vi "FeedbackDecode_BuildStimCmd.vi"(2 "EncodeClustIn":T1={"ParamsTable"=[], "Sel"=[], "Stim"=FALSE, "StimMode"=enum."Off", "StimStep"=[enum."1uA", enum."1uA", enum."Off"], "Jitter"=FALSE, "Pulse"=FALSE, "BFreq"=0.0, "BAmp"=0.0, "UEAArray"=[], "AdjClust"={"Add"=FALSE, "Sub"=FALSE, "Val"=[1.0, 100.0, 0.2, 500.0, 0.0], "B"=[FALSE, FALSE, FALSE, FALSE, FALSE], "Inc+"=["x+1", "x+10", "x+0.1", "x+10", "x+10"], "Set"=FALSE, "LoadTable"=FALSE, "SaveTable"=FALSE, "ClearTable"=FALSE, "DeleteSel"=FALSE, "Inc-"=["x-1", "x-10", "x-0.1", "x-10", "x-10"]}, "PresetTable"=[], "SelPreset"=[], "SortClust"={"Region"=FALSE, "Receptor"=FALSE, "Electrode"=FALSE, "Min Amp"=FALSE, "Max Amp"=FALSE, "Min Freq"=FALSE, "Max Freq"=FALSE, "Duration"=FALSE}, "SelSort"={"Sel"=FALSE}, "PresetClust"={"Load"=FALSE, "Clear"=FALSE, "Save"=FALSE, "Del"=FALSE}, "RespClust"={"RespType"=enum."Sensor Map", "OpenResp"=FALSE}, "AmpLimit"=0.0, "FreqLimit"=0.0, "DurLimit"=0.0, "Wait Period"=0.0, "Train Period"=0.0} {"Train Period" min=0.0 max=100.0 step=0.1; "Wait Period" min=0.0 max=100.0 step=0.1; "DurLimit" min=0.0 max=1.0 step=0.01; "FreqLimit" min=0.0 max=500.0 step=1.0; "AmpLimit" min=0.0 max=100.0 step=1.0; "BAmp" min=0.0 max=100.0 step=1.0; "BFreq" min=0.0 max=100.0 step=1.0}) -> (0 "EncodeClustOut":T1={"ParamsTable"=[], "Sel"=[], "Stim"=FALSE, "StimMode"=enum."Off", "StimStep"=[enum."1uA", enum."1uA", enum."Off"], "Jitter"=FALSE, "Pulse"=FALSE, "BFreq"=0.0, "BAmp"=0.0, "UEAArray"=[], "AdjClust"={"Add"=FALSE, "Sub"=FALSE, "Val"=[1.0, 100.0, 0.2, 500.0, 0.0], "B"=[FALSE, FALSE, FALSE, FALSE, FALSE], "Inc+"=["x+1", "x+10", "x+0.1", "x+10", "x+10"], "Set"=FALSE, "LoadTable"=FALSE, "SaveTable"=FALSE, "ClearTable"=FALSE, "DeleteSel"=FALSE, "Inc-"=["x-1", "x-10", "x-0.1", "x-10", "x-10"]}, "PresetTable"=[], "SelPreset"=[], "SortClust"={"Region"=FALSE, "Receptor"=FALSE, "Electrode"=FALSE, "Min Amp"=FALSE, "Max Amp"=FALSE, "Min Freq"=FALSE, "Max Freq"=FALSE, "Duration"=FALSE}, "SelSort"={"Sel"=FALSE}, "PresetClust"={"Load"=FALSE, "Clear"=FALSE, "Save"=FALSE, "Del"=FALSE}, "RespClust"={"RespType"=enum."Sensor Map", "OpenResp"=FALSE}, "AmpLimit"=0.0, "FreqLimit"=0.0, "DurLimit"=0.0, "Wait Period"=0.0, "Train Period"=0.0} {"Train Period" min=0.0 max=100.0 step=0.1; "Wait Period" min=0.0 max=100.0 step=0.1; "DurLimit" min=0.0 max=1.0 step=0.01; "FreqLimit" min=0.0 max=500.0 step=1.0; "AmpLimit" min=0.0 max=100.0 step=1.0; "BAmp" min=0.0 max=100.0 step=1.0; "BFreq" min=0.0 max=100.0 step=1.0}, 1 "StimCmd":string)   [LabVIEW 2020]
uses:
  FeedbackDecode_EncodeClust.ctl
  FeedbackDecode_VariablesToString_Array.vi
  FeedbackDecode_VariablesToString_Scalar.vi
panel:
  in  "Receptor":string[](array[string])=["MS1", "MS2", "SA1", "RA1", "RA2", "aSA", "aRA", "scaled", "bio amp", "bio freq", "proprio"]
  in  "Region":string[](array[string])=["thumb_distal", "thumb_medial", "thumb_proximal", "index_distal", "index_medial", "index_proximal", "middle_distal", "middle_medial", "middle_proximal", "ring_distal", "ring_medial", "ring_proximal", "pinky_distal", "pinky_medial", "pinky_proximal", "palm_back", "palm_side", "palm_pinky", "palm_thumb", "thumb_MCP", "thumb_PIP", "thumb_DIP", "thumb_ABD", "index_MCP", "index_ABD", "middle_MCP", "ring_MCP", "pinky_MCP", "pinky_ABD", "wrist_FLEX", "wrist_UDEV", "wrist_PRO"]
  # "Value"
  # "Inc-"
  # "Inc+"
  # "Min Amp"
  # "Max Amp"
  # "Min Freq"
  # "Max Freq"
  # "Duration"
  # "Value"
  # "Inc-"
  # "Inc+"
  # "Min Amp"
  # "Max Amp"
  # "Min Freq"
  # "Max Freq"
  # "Duration"
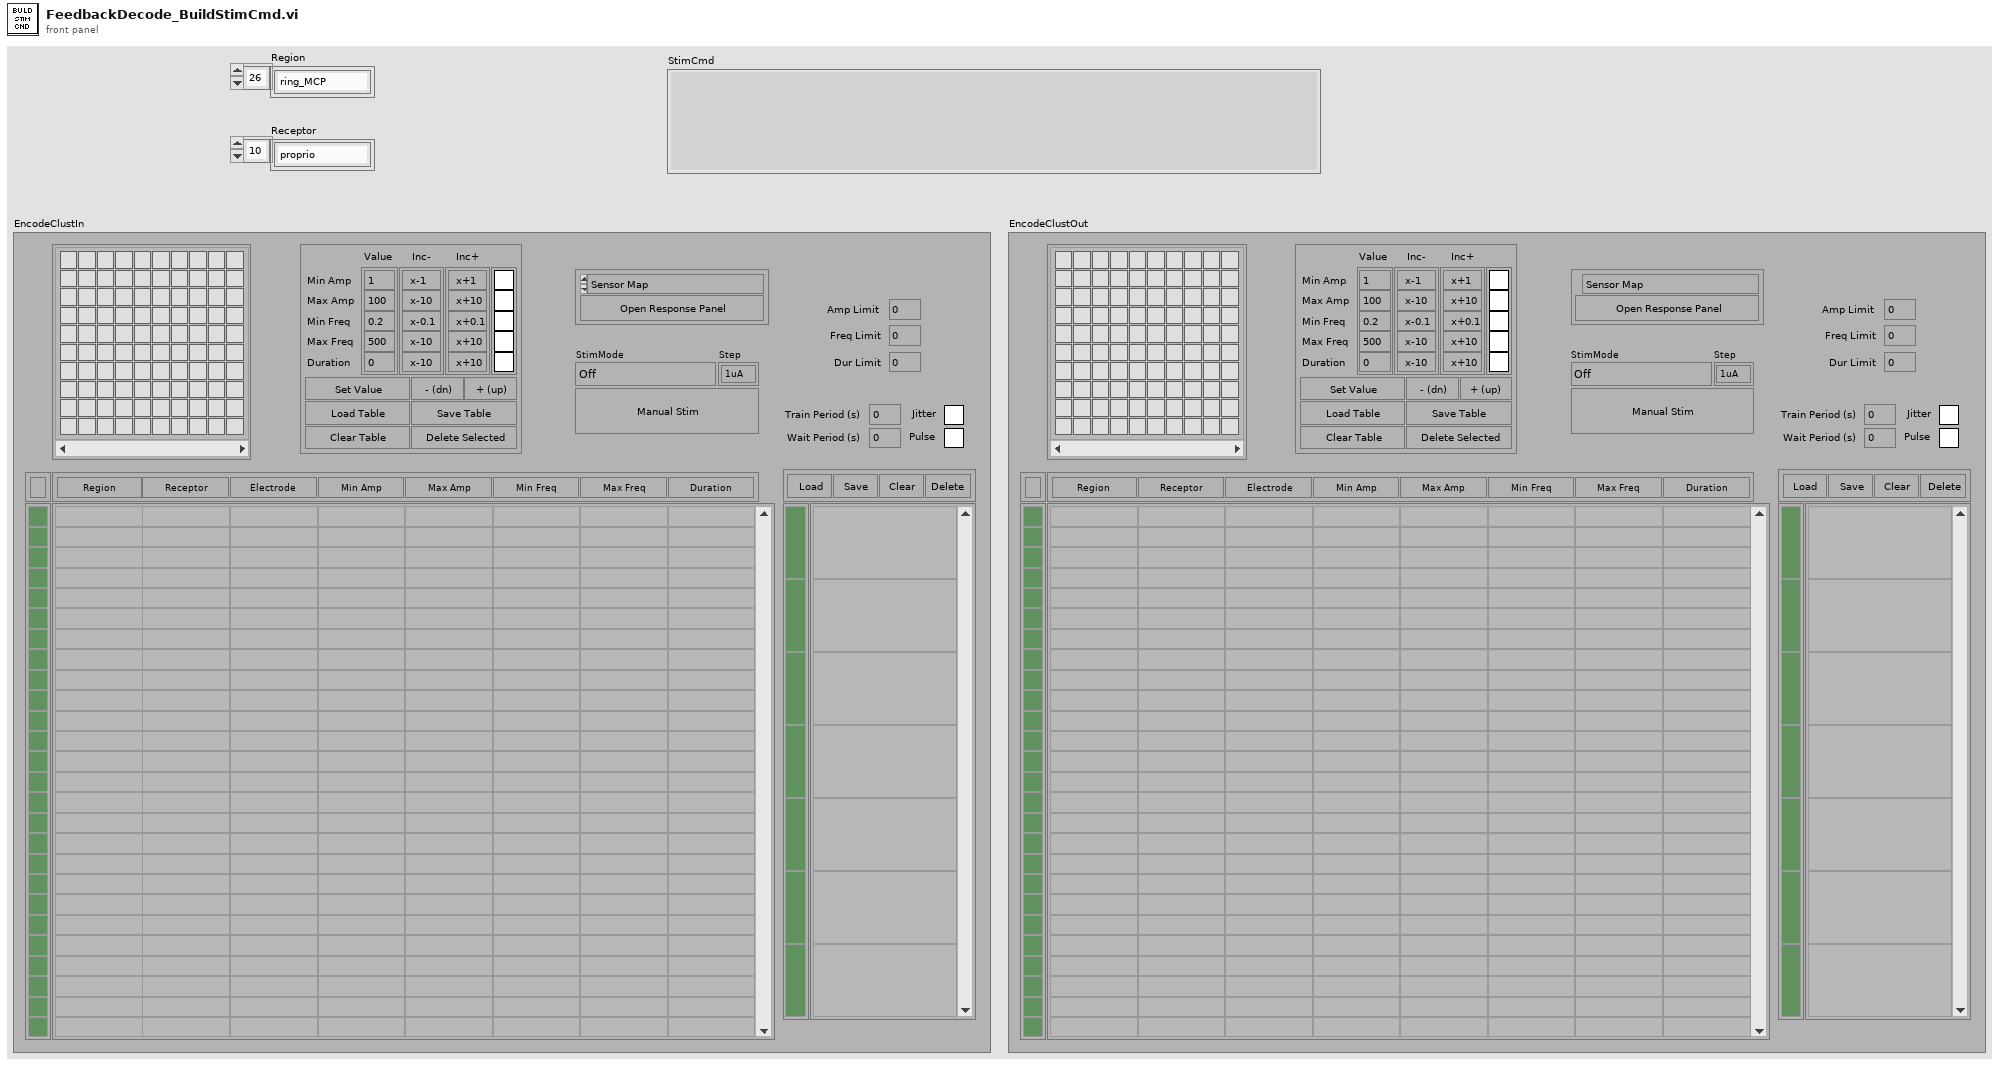
[diagram p1: front panel]
types:
  T1 = typedef "FeedbackDecode_EncodeClust.ctl" = cluster{"ParamsTable":string[][], "Sel":bool[], "Stim":bool, "StimMode":enum16{"Off", "Manual", "MSMS", "VRE", "3DHand", "DEKA", "Analog(DEKA)"}, "StimStep":enum16{"Off", "1uA", "2uA", "5uA", "10uA", "20uA", "30uA"}[], "Jitter":bool, "Pulse":bool, "BFreq":dbl, "BAmp":dbl, "UEAArray":cluster{"Boolean 1":bool, "Boolean 2":bool, "Boolean 3":bool, "Boolean 4":bool, "Boolean 5":bool, "Boolean 6":bool, "Boolean 7":bool, "Boolean 8":bool, "Boolean 9":bool, "Boolean 10":bool, "Boolean 11":bool, "Boolean 12":bool, "Boolean 13":bool, "Boolean 14":bool, "Boolean 15":bool, "Boolean 16":bool, "Boolean 17":bool, "Boolean 18":bool, "Boolean 19":bool, "Boolean 20":bool, "Boolean 21":bool, "Boolean 22":bool, "Boolean 23":bool, "Boolean 24":bool, "Boolean 25":bool, "Boolean 26":bool, "Boolean 27":bool, "Boolean 28":bool, "Boolean 29":bool, "Boolean 30":bool, "Boolean 31":bool, "Boolean 32":bool, "Boolean 33":bool, "Boolean 34":bool, "Boolean 35":bool, "Boolean 36":bool, "Boolean 37":bool, "Boolean 38":bool, "Boolean 39":bool, "Boolean 40":bool, "Boolean 41":bool, "Boolean 42":bool, "Boolean 43":bool, "Boolean 44":bool, "Boolean 45":bool, "Boolean 46":bool, "Boolean 47":bool, "Boolean 48":bool, "Boolean 49":bool, "Boolean 50":bool, "Boolean 51":bool, "Boolean 52":bool, "Boolean 53":bool, "Boolean 54":bool, "Boolean 55":bool, "Boolean 56":bool, "Boolean 57":bool, "Boolean 58":bool, "Boolean 59":bool, "Boolean 60":bool, "Boolean 61":bool, "Boolean 62":bool, "Boolean 63":bool, "Boolean 64":bool, "Boolean 65":bool, "Boolean 66":bool, "Boolean 67":bool, "Boolean 68":bool, "Boolean 69":bool, "Boolean 70":bool, "Boolean 71":bool, "Boolean 72":bool, "Boolean 73":bool, "Boolean 74":bool, "Boolean 75":bool, "Boolean 76":bool, "Boolean 77":bool, "Boolean 78":bool, "Boolean 79":bool, "Boolean 80":bool, "Boolean 81":bool, "Boolean 82":bool, "Boolean 83":bool, "Boolean 84":bool, "Boolean 85":bool, "Boolean 86":bool, "Boolean 87":bool, "Boolean 88":bool, "Boolean 89":bool, "Boolean 90":bool, "Boolean 91":bool, "Boolean 92":bool, "Boolean 93":bool, "Boolean 94":bool, "Boolean 95":bool, "Boolean 96":bool, "Boolean 97":bool, "Boolean 98":bool, "Boolean 99":bool, "Boolean 100":bool}[], "AdjClust":cluster{"Add":bool, "Sub":bool, "Val":dbl[], "B":bool[], "Inc+":string[], "Set":bool, "LoadTable":bool, "SaveTable":bool, "ClearTable":bool, "DeleteSel":bool, "Inc-":string[]}, "PresetTable":string[][], "SelPreset":bool[], "SortClust":cluster{"Region":bool, "Receptor":bool, "Electrode":bool, "Min Amp":bool, "Max Amp":bool, "Min Freq":bool, "Max Freq":bool, "Duration":bool}, "SelSort":cluster{"Sel":bool}, "PresetClust":cluster{"Load":bool, "Clear":bool, "Save":bool, "Del":bool}, "RespClust":cluster{"RespType":enum16{"Sensor Map", "Full Map"}, "OpenResp":bool}, "AmpLimit":dbl, "FreqLimit":dbl, "DurLimit":dbl, "Wait Period":dbl, "Train Period":dbl}
  T2 = enum16{"Off", "Manual", "MSMS", "VRE", "3DHand", "DEKA", "Analog(DEKA)"}
  T3 = enum16{"Off", "1uA", "2uA", "5uA", "10uA", "20uA", "30uA"}[]
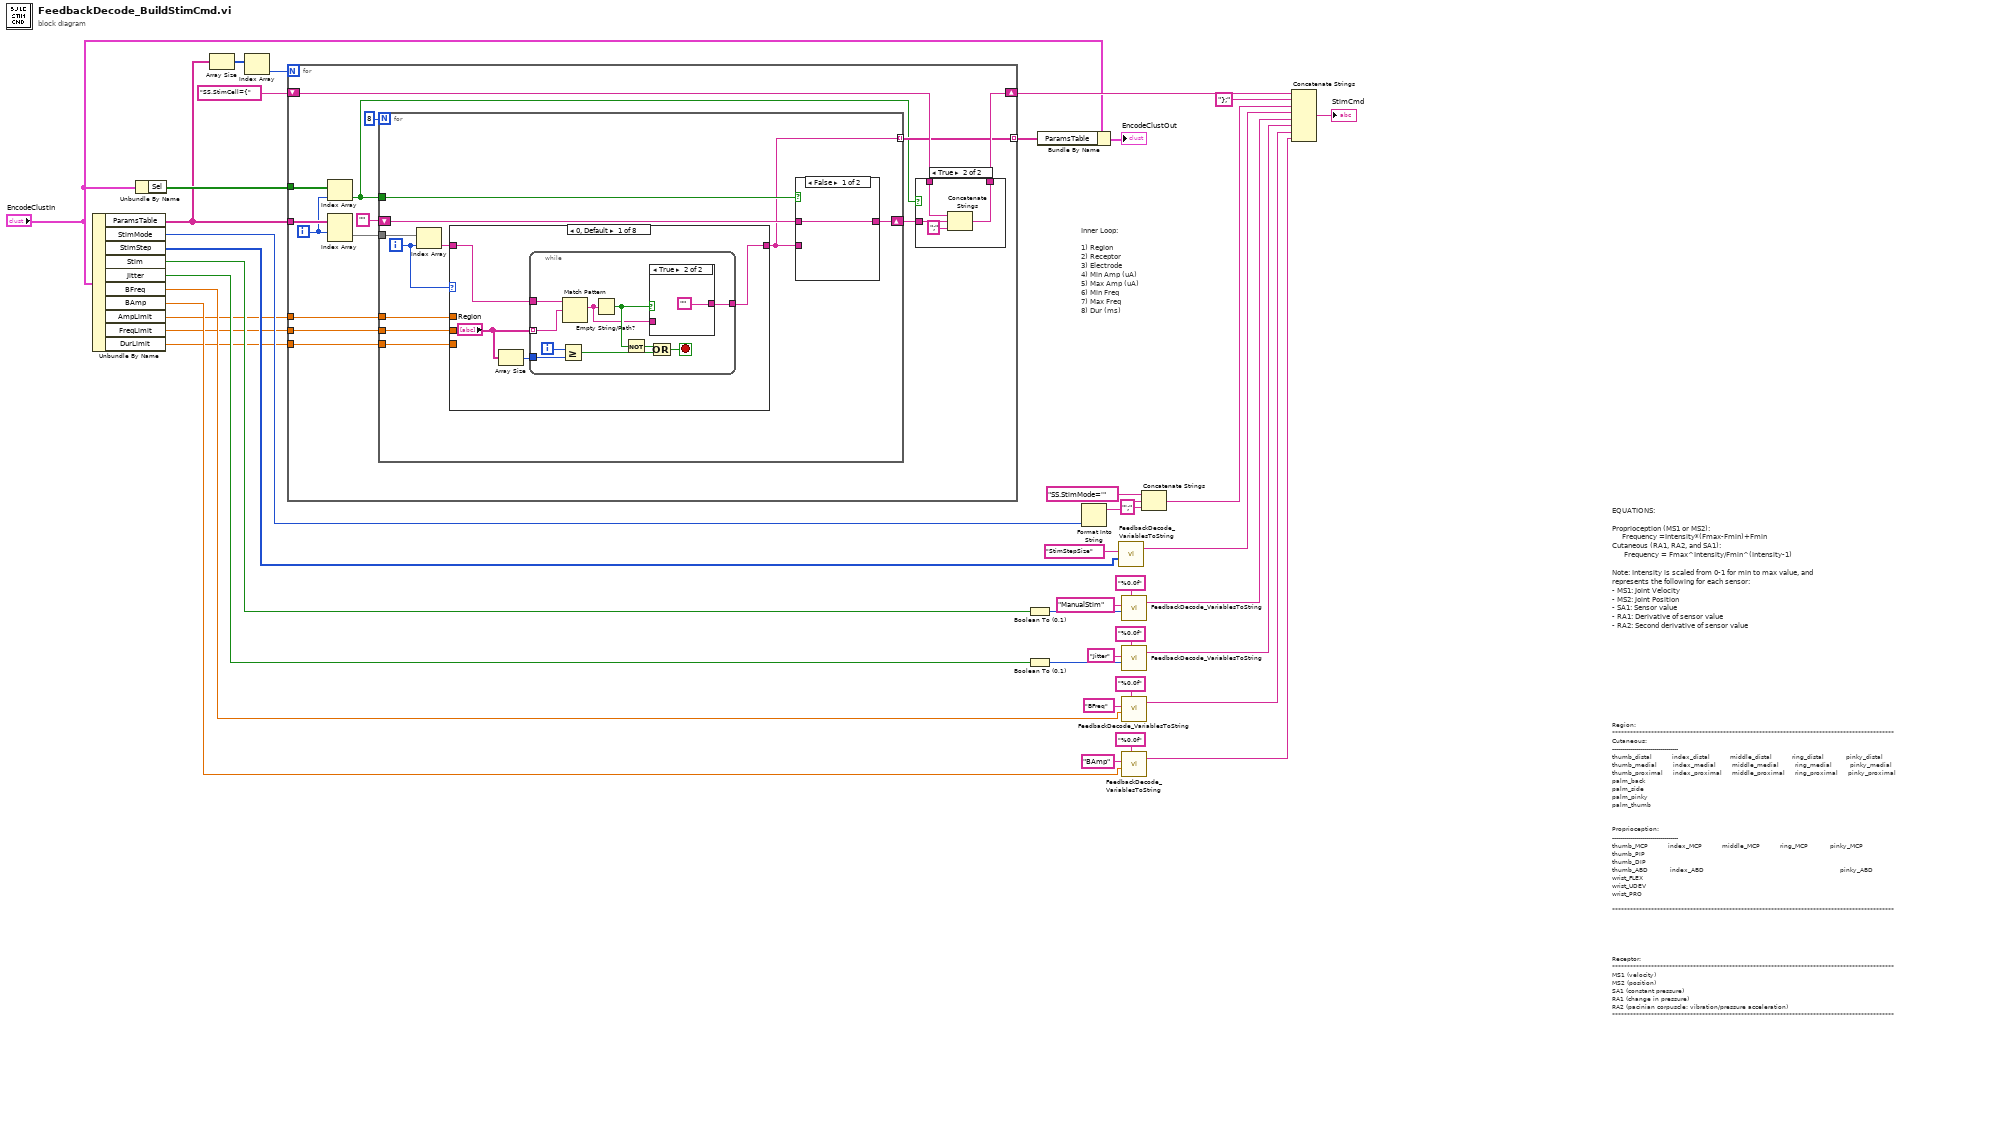
[diagram p0: block diagram]
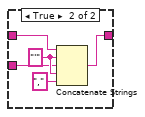
[diagram p3: hidden frame]
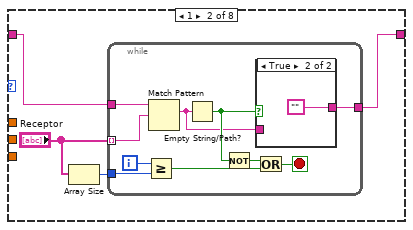
[diagram p5: hidden frame]
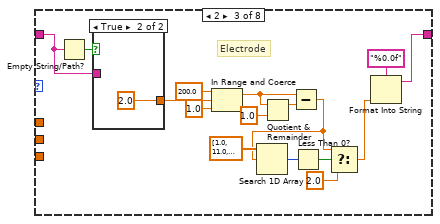
[diagram p7: hidden frame]
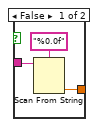
[diagram p8: hidden frame]
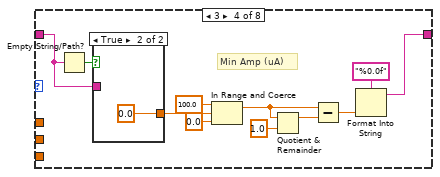
[diagram p9: hidden frame]
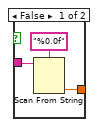
[diagram p10: hidden frame]
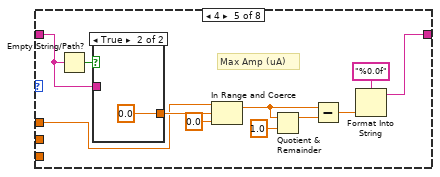
[diagram p11: hidden frame]
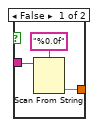
[diagram p12: hidden frame]
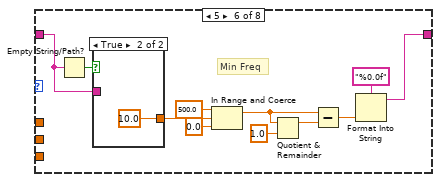
[diagram p13: hidden frame]
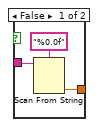
[diagram p14: hidden frame]
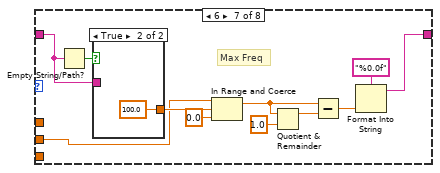
[diagram p15: hidden frame]
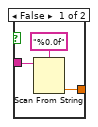
[diagram p16: hidden frame]
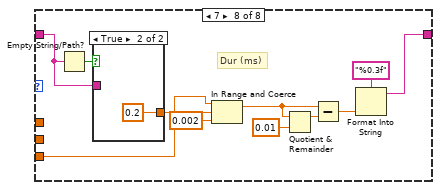
[diagram p17: hidden frame]
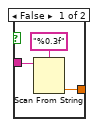
[diagram p18: hidden frame]
diagram:
  # "Inner Loop:\n\n1) Region\n2) Receptor\n3) Electrode\n4) Min Amp (uA)\n5) Max Amp (uA)\n6) Min Freq\n7) Max Freq\n8) Dur (ms)"
  # "EQUATIONS:\n\nProprioception (MS1 or MS2):\n     Frequency =Intensity*(Fmax-Fmin)+Fmin\nCutaneous (RA1, RA2, and SA1):     \n      Frequency = Fmax^Intensity/Fmin^(Intensity-1)\n\nNote: Intensity is scaled from 0-1 for min to max value, and represents the following for each sensor:\n- MS1: Joint Velocity\n- MS2: Joint Position\n- SA1: Sensor value\n- RA1: Derivative of sensor value\n- RA2: Second derivative of sensor value"
  # "Region:\n**********************************************************************************************\nCutaneous:\n---------------------------------\nthumb_distal          index_distal          middle_distal          ring_distal           pinky_distal\nthumb_medial        index_medial        middle_medial        ring_medial         pinky_medial\nthumb_proximal     index_proximal     middle_proximal     ring_proximal     pinky_proximal\npalm_back\npalm_side\npalm_pinky\npalm_thumb\n\n\nProprioception:\n---------------------------------\nthumb_MCP          index_MCP          middle_MCP          ring_MCP           pinky_MCP\nthumb_PIP                          \nthumb_DIP                                   \nthumb_ABD           index_ABD                                                                    pinky_ABD\nwrist_FLEX\nwrist_UDEV\nwrist_PRO\n\n**********************************************************************************************\n\n\n\n\n\nReceptor:\n**********************************************************************************************\nMS1 (velocity)\nMS2 (position)\nSA1 (constant pressure)\nRA1 (change in pressure)\nRA2 (pacinian corpuscle: vibration/pressure acceleration)\n**********************************************************************************************"
  n1 = Unbundle By Name("EncodeClustIn") -> ("ParamsTable"=w34:string[][], "StimMode"=w27:T2, "StimStep"=w26:T3, "Stim"=w18:bool, "Jitter"=w13:bool, "BFreq"=w9:dbl, "BAmp"=w5:dbl, "AmpLimit"=w3:dbl, "FreqLimit"=w2:dbl, "DurLimit"=w1:dbl)
  n2 = Unbundle By Name("EncodeClustIn") -> ("Sel"=w40:bool[])
  n3 = Array Size(array=w34) -> (size(s)=w33:i32[])
  n4 = Index Array(array=w33) -> (element=w32:i32)  [unwired: 1 in]
  n5 = for {
    N: w32 -> [_]
    tunnel: w40 -> [w46]
    tunnel: w34 -> [w48]
    shift-right: [w53] -> w39
    shift-left: "SS.StimCell={" -> [w54]
    tunnel: [w47] -> w36 mode=indexing
    tunnel: w3 -> [w43]
    tunnel: w2 -> [w42]
    tunnel: w1 -> [w41]
    i -> [w45]
    n6 = Index Array(array=w46, index=w45) -> (element=w44:bool)
    n7 = Index Array(array=w48, index (row)=w45) -> (element=w51:string[])  [unwired: 1 in]
    n8 = for {
      N: 8 -> [_]
      tunnel: w51 -> [w69]
      shift-right: [w67] -> w49
      shift-left: "" -> [w68]
      tunnel: w44 -> [w65]
      tunnel: [w63] -> w47 mode=indexing
      tunnel: w43 -> [w62]
      tunnel: w42 -> [w61]
      tunnel: w41 -> [w60]
      i -> [w64]
      n9 = Index Array(array=w69, index=w64) -> (element=w66:string)
      n10 = case shown="0, Default" w64 {
        tunnel: w66 -> [w79 w94 w114 w129 w145 w159 w175 w189]
        tunnel: [w78 w93 w116 w128 w144 w158 w174 w190] -> w63
        tunnel: w62 -> [_ _ _ _ w143 _ _ _]
        tunnel: w61 -> [_ _ _ _ _ _ w173 _]
        tunnel: w60 -> [_ _ _ _ _ _ _ w188]
        frame 0, Default {
          n11 = Array Size(array="Region") -> (size(s)=w77:i32)
          n12 = while {
            tunnel: "Region" -> [w88] mode=indexing
            tunnel: w79 -> [w89]
            tunnel: [w80] -> w78
            tunnel: w77 -> [w87]
            i -> [w86]
            stop <- w83 stop-if-true
            n13 = Greater Or Equal?(x=w86, y=w87) -> (x >= y?=w84:bool)
            n14 = Match Pattern(string=w89, regular expression=w88) -> (match substring=w81:string)  [unwired: 1 in, 3 out]
            n15 = Empty String/Path?(string/path=w81) -> (empty?=w82:bool)
            n16 = Not(x=w82) -> (.not. x?=w85:bool)
            n17 = case shown="True" w82 {
              tunnel: w81 -> [w90 _]
              tunnel: [w90 ""] -> w80
              frame False {
              }
              frame True {
              }
            }
            n18 = Or(x=w85, y=w84) -> (x .or. y?=w83:bool)
          }
        }
        frame 1 {
          n19 = Array Size(array="Receptor") -> (size(s)=w95:i32)
          n20 = while {
            tunnel: "Receptor" -> [w104] mode=indexing
            tunnel: w94 -> [w105]
            tunnel: [w96] -> w93
            tunnel: w95 -> [w103]
            i -> [w102]
            stop <- w99 stop-if-true
            n21 = Greater Or Equal?(x=w102, y=w103) -> (x >= y?=w100:bool)
            n22 = Match Pattern(string=w105, regular expression=w104) -> (match substring=w97:string)  [unwired: 1 in, 3 out]
            n23 = Empty String/Path?(string/path=w97) -> (empty?=w98:bool)
            n24 = Not(x=w98) -> (.not. x?=w101:bool)
            n25 = case shown="True" w98 {
              tunnel: w97 -> [w106 _]
              tunnel: [w106 ""] -> w96
              frame False {
              }
              frame True {
              }
            }
            n26 = Or(x=w101, y=w100) -> (x .or. y?=w99:bool)
          }
        }
        frame 2 {
          # "Electrode"
          n27 = Empty String/Path?(string/path=w114) -> (empty?=w115:bool)
          n28 = case shown="True" w115 {
            tunnel: [w125 2.0] -> w117
            tunnel: w114 -> [w124 _]
            frame False {
              n29 = Scan From String(format string="%0.0f", input string=w124) -> (output 1=w125:dbl)  [unwired: 3 in, 3 out]
            }
            frame True {
            }
          }
          n30 = In Range and Coerce(upper limit=200.0, x=w117, lower limit=1.0) -> (coerced(x)=w123:dbl)  [unwired: 1 out]
          n31 = Quotient & Remainder(x=w123, y=1.0) -> (x-y*floor(x/y)=w120:dbl)  [unwired: 1 out]
          n32 = Subtract(x=w123, y=w120) -> (x-y=w110:dbl)
          n33 = Search 1D Array(1D array=dbl[] [1.0, 11.0, 81.0, 91.0, 101.0, 111.0, 181.0, 191.0], element=w110) -> (index of element=w111:i32)  [unwired: 1 in]
          n34 = Less Than 0?(x=w111) -> (x < 0?=w112:bool)
          n35 = Select(t=w110, s=w112, f=2.0) -> (s? t:f=w109:dbl)
          n36 = Format Into String(format string="%0.0f", w109) -> (resulting string=w116:string)  [unwired: 2 in, 1 out]
        }
        frame 3 {
          # "Min Amp (uA)"
          n37 = Empty String/Path?(string/path=w129) -> (empty?=w130:bool)
          n38 = case shown="True" w130 {
            tunnel: [w140 0.0] -> w132
            tunnel: w129 -> [w139 _]
            frame False {
              n39 = Scan From String(format string="%0.0f", input string=w139) -> (output 1=w140:dbl)  [unwired: 3 in, 3 out]
            }
            frame True {
            }
          }
          n40 = In Range and Coerce(upper limit=100.0, x=w132, lower limit=0.0) -> (coerced(x)=w138:dbl)  [unwired: 1 out]
          n41 = Quotient & Remainder(x=w138, y=1.0) -> (x-y*floor(x/y)=w135:dbl)  [unwired: 1 out]
          n42 = Subtract(x=w138, y=w135) -> (x-y=w131:dbl)
          n43 = Format Into String(format string="%0.0f", w131) -> (resulting string=w128:string)  [unwired: 2 in, 1 out]
        }
        frame 4 {
          # "Max Amp (uA)"
          n44 = Empty String/Path?(string/path=w145) -> (empty?=w146:bool)
          n45 = case shown="True" w146 {
            tunnel: [w155 0.0] -> w148
            tunnel: w145 -> [w154 _]
            frame False {
              n46 = Scan From String(format string="%0.0f", input string=w154) -> (output 1=w155:dbl)  [unwired: 3 in, 3 out]
            }
            frame True {
            }
          }
          n47 = In Range and Coerce(upper limit=w143, x=w148, lower limit=0.0) -> (coerced(x)=w153:dbl)  [unwired: 1 out]
          n48 = Quotient & Remainder(x=w153, y=1.0) -> (x-y*floor(x/y)=w151:dbl)  [unwired: 1 out]
          n49 = Subtract(x=w153, y=w151) -> (x-y=w147:dbl)
          n50 = Format Into String(format string="%0.0f", w147) -> (resulting string=w144:string)  [unwired: 2 in, 1 out]
        }
        frame 5 {
          # "Min Freq"
          n51 = Empty String/Path?(string/path=w159) -> (empty?=w160:bool)
          n52 = case shown="True" w160 {
            tunnel: [w170 10.0] -> w162
            tunnel: w159 -> [w169 _]
            frame False {
              n53 = Scan From String(format string="%0.0f", input string=w169) -> (output 1=w170:dbl)  [unwired: 3 in, 3 out]
            }
            frame True {
            }
          }
          n54 = In Range and Coerce(upper limit=500.0, x=w162, lower limit=0.0) -> (coerced(x)=w168:dbl)  [unwired: 1 out]
          n55 = Quotient & Remainder(x=w168, y=1.0) -> (x-y*floor(x/y)=w165:dbl)  [unwired: 1 out]
          n56 = Subtract(x=w168, y=w165) -> (x-y=w161:dbl)
          n57 = Format Into String(format string="%0.0f", w161) -> (resulting string=w158:string)  [unwired: 2 in, 1 out]
        }
        frame 6 {
          # "Max Freq"
          n58 = Empty String/Path?(string/path=w175) -> (empty?=w176:bool)
          n59 = case shown="True" w176 {
            tunnel: [w185 100.0] -> w178
            tunnel: w175 -> [w184 _]
            frame False {
              n60 = Scan From String(format string="%0.0f", input string=w184) -> (output 1=w185:dbl)  [unwired: 3 in, 3 out]
            }
            frame True {
            }
          }
          n61 = In Range and Coerce(upper limit=w173, x=w178, lower limit=0.0) -> (coerced(x)=w183:dbl)  [unwired: 1 out]
          n62 = Quotient & Remainder(x=w183, y=1.0) -> (x-y*floor(x/y)=w181:dbl)  [unwired: 1 out]
          n63 = Subtract(x=w183, y=w181) -> (x-y=w177:dbl)
          n64 = Format Into String(format string="%0.0f", w177) -> (resulting string=w174:string)  [unwired: 2 in, 1 out]
        }
        frame 7 {
          # "Dur (ms)"
          n65 = Empty String/Path?(string/path=w189) -> (empty?=w191:bool)
          n66 = case shown="True" w191 {
            tunnel: [w200 0.2] -> w193
            tunnel: w189 -> [w199 _]
            frame False {
              n67 = Scan From String(format string="%0.3f", input string=w199) -> (output 1=w200:dbl)  [unwired: 3 in, 3 out]
            }
            frame True {
            }
          }
          n68 = In Range and Coerce(upper limit=w188, x=w193, lower limit=0.002) -> (coerced(x)=w198:dbl)  [unwired: 1 out]
          n69 = Quotient & Remainder(x=w198, y=0.01) -> (x-y*floor(x/y)=w196:dbl)  [unwired: 1 out]
          n70 = Subtract(x=w198, y=w196) -> (x-y=w192:dbl)
          n71 = Format Into String(format string="%0.3f", w192) -> (resulting string=w190:string)  [unwired: 2 in, 1 out]
        }
      }
      n72 = case shown="False" w65 {
        tunnel: w68 -> [w70 w73]
        tunnel: [w70 w72] -> w67
        tunnel: w63 -> [_ w71]
        frame False {
        }
        frame True {
          w75 = "'" ("string")
          n73 = Concatenate Strings(w73, w75, w71, w75, "," ("string")) -> (w72:string)
        }
      }
    }
    n74 = case shown="True" w44 {
      tunnel: w54 -> [w55 w59]
      tunnel: [w55 w58] -> w53
      tunnel: w49 -> [_ w57]
      frame False {
      }
      frame True {
        n75 = Concatenate Strings(w59, w57, ";" ("string")) -> (w58:string)
      }
    }
  }
  n76 = Boolean To (0,1)(Boolean=w18) -> (0, 1=w19:i16)
  n77 = Boolean To (0,1)(Boolean=w13) -> (0, 1=w16:i16)
  n78 = Bundle By Name(cluster="EncodeClustIn", "ParamsTable"=w36) -> (→"EncodeClustOut":T1)
  n79 = Format Into String(w27) -> (resulting string=w30:string)  [unwired: 3 in, 1 out]
  n80 = call-poly "FeedbackDecode_VariablesToString.vi"("ValueIn"=w26, "FieldName"="StimStepSize") -> ("StringOut"=w24:string)  [unwired: 5 in]
  n81 = call-poly "FeedbackDecode_VariablesToString.vi"("Format"="%0.0f", "ValueIn"=w19, "FieldName"="ManualStim") -> ("StringOut"=w17:string)  [unwired: 4 in]
  n82 = call-poly "FeedbackDecode_VariablesToString.vi"("Format"="%0.0f", "ValueIn"=w16, "FieldName"="Jitter") -> ("StringOut"=w12:string)  [unwired: 4 in]
  n83 = call-poly "FeedbackDecode_VariablesToString.vi"("Format"="%0.0f", "ValueIn"=w9, "FieldName"="BFreq") -> ("StringOut"=w8:string)  [unwired: 4 in]
  n84 = call-poly "FeedbackDecode_VariablesToString.vi"("Format"="%0.0f", "ValueIn"=w5, "FieldName"="BAmp") -> ("StringOut"=w4:string)  [unwired: 4 in]
  n85 = Concatenate Strings("SS.StimMode='" ("string"), w30, "';" ("string")) -> (w25:string)
  n86 = Concatenate Strings(w39, "};" ("string"), w25, w24, w17, w12, w8, w4) -> (→"StimCmd":string)
